vi "(SubVI)_2D_CreateFile_MultiVessel_Ver17.vi"(2 "Scanning Method":enum16{"2D", "3D"}(ring), 4 "B-scan Rep":dbl, 6 "error in":errorcluster, 7 "2D Label":string="Untitled", 8 "BD":bool=TRUE, 9 "Camera Param":T2, 10 "Galvo Param":T1, 11 "Path":path=path "C:/OCT_Data") -> (0 "error out":errorcluster, 3 "refnum out":refnum<file>)   [LabVIEW 2019]
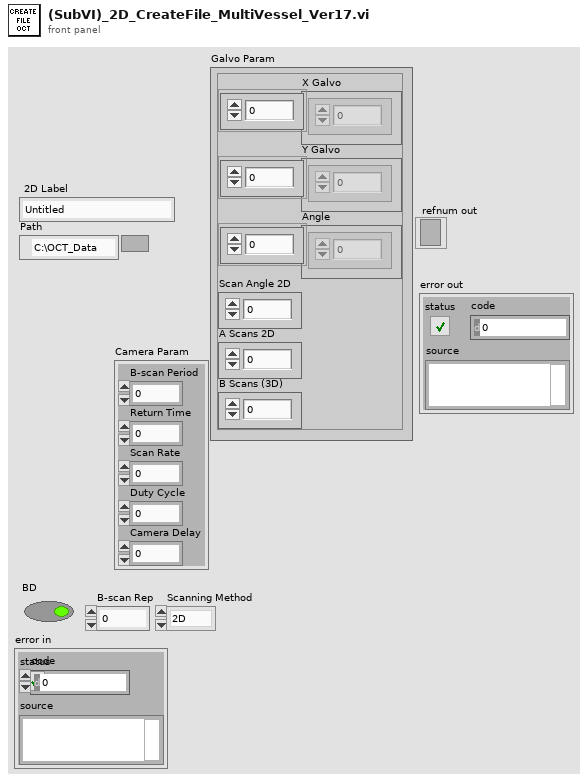
[diagram p1: front panel]
types:
  T1 = cluster{"X Galvo":dbl[], "Y Galvo":dbl[], "Angle":dbl[], "Scan Angle 2D":dbl, "A Scans 2D":u32, "B Scans (3D)":u32}
  T2 = cluster{"B-scan Period":dbl, "Return Time":dbl, "Scan Rate":dbl, "Duty Cycle":dbl, "Camera Delay":dbl}
  T3 = enum16{"big-endian, network order", "native, host order", "little-endian"}
  T4 = enum16{"open", "replace", "create", "open or create", "replace or create", "replace or create with confirmation"}
  T5 = cluster{"string":string, "string":string, "string":string, "Scan Angle 2D":dbl, "string":string, "X Galvo":dbl[], "string":string, "Y Galvo":dbl[], "string":string, "Angle":dbl[], "string":string, "Scan Angle 2D":dbl, "string":string, dbl, "string":string, dbl}
  T6 = cluster{"string":string, "B-scan Period":dbl, "string":string, "Return Time":dbl, "string":string, "Scan Rate":dbl, "string":string, "Camera Delay":dbl, "string":string, "Duty Cycle":dbl, "string":string, "Scan Rate":dbl}
  T7 = cluster{cluster{"string":string, "string":string, "string":string, "Scan Angle 2D":dbl, "string":string, "X Galvo":dbl[], "string":string, "Y Galvo":dbl[], "string":string, "Angle":dbl[], "string":string, "Scan Angle 2D":dbl, "string":string, dbl, "string":string, dbl}, cluster{"string":string, "B-scan Period":dbl, "string":string, "Return Time":dbl, "string":string, "Scan Rate":dbl, "string":string, "Camera Delay":dbl, "string":string, "Duty Cycle":dbl, "string":string, "Scan Rate":dbl}, cluster{"string":string, "B-scan Rep":dbl}, "string":string, "string":string}
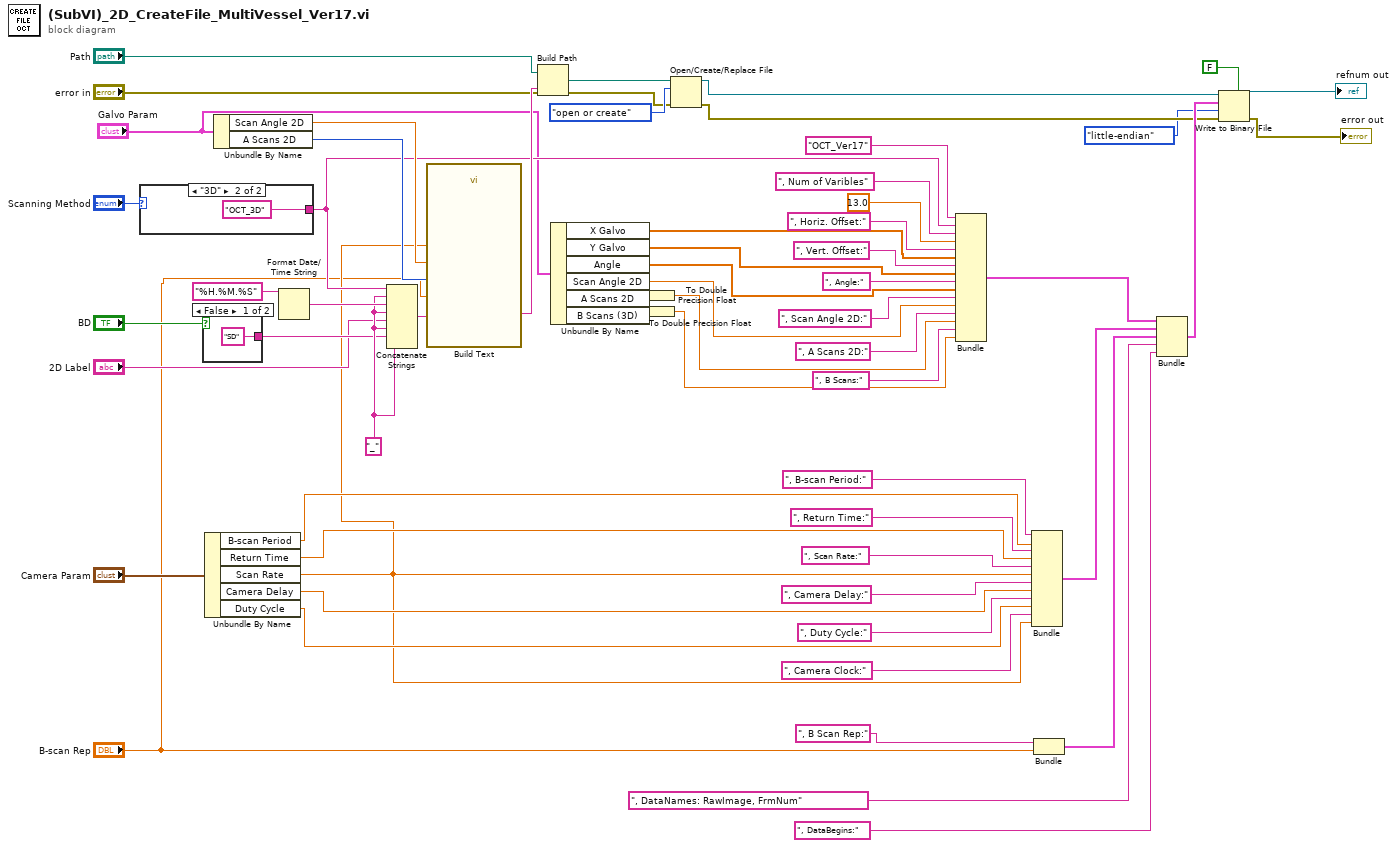
[diagram p0: block diagram]
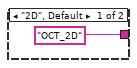
[diagram p2: hidden frame]
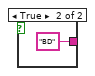
[diagram p3: hidden frame]
diagram:
  w55 = "_" ("3D Label")
  n1 = case shown="\"3D\"" "Scanning Method" {
    tunnel: ["OCT_2D" ("string") "OCT_3D" ("string")] -> w11
    frame "2D", Default {
    }
    frame "3D" {
    }
  }
  n2 = case shown="False" "BD" {
    tunnel: ["SD" ("string") "BD" ("string")] -> w53
    frame False {
    }
    frame True {
    }
  }
  n3 = Unbundle By Name("Camera Param") -> ("B-scan Period"=w9:dbl, "Return Time"=w8:dbl, "Scan Rate"=w5:dbl, "Camera Delay"=w7:dbl, "Duty Cycle"=w6:dbl)
  n4 = Unbundle By Name("Galvo Param") -> ("Scan Angle 2D"=w48:dbl, "A Scans 2D"=w52:u32)
  n5 = Format Date/Time String(time format string (%c)="%H.%M.%S") -> (date/time string=w59:string)  [unwired: 2 in]
  n6 = Concatenate Strings(w11, w55, w59, w55, "2D Label", w55, w53, w55) -> (w58:string)
  n7 = call "Build Text"("Beginning Text"=w58, "x"="B-scan Rep", "K"=w5, "SA"=w48, "A"=w52) -> ("Result"=w57:string)  [unwired: 9 in, 1 out]
  n8 = Build Path(base path="Path", name or relative path=w57) -> (appended path=w50:path)
  n9 = Unbundle By Name("Galvo Param") -> ("X Galvo"=w14:dbl[], "Y Galvo"=w13:dbl[], "Angle"=w15:dbl[], "Scan Angle 2D"=w16:dbl, "A Scans 2D"=w46:u32, "B Scans (3D)"=w22:u32)
  n10 = To Double Precision Float(number=w46) -> (double precision float=w40:dbl)
  n11 = To Double Precision Float(number=w22) -> (double precision float=w21:dbl)
  n12 = Open/Create/Replace File(file path (use dialog)=w50, error in="error in", operation (0:open)=T4."open or create") -> (refnum out=w30:refnum<file>, error out=w29:errorcluster)  [unwired: 3 in, 1 out]
  n13 = Bundle("string"="OCT_Ver17", "string"=w11, "string"=", Num of Varibles", "Scan Angle 2D"=13.0, "string"=", Horiz. Offset:", "X Galvo"=w14, "string"=", Vert. Offset:", "Y Galvo"=w13, "string"=", Angle:", "Angle"=w15, "string"=", Scan Angle 2D:", "Scan Angle 2D"=w16, "string"=", A Scans 2D:", w40, "string"=", B Scans:", w21) -> (w33:T5)  [unwired: 1 in]
  n14 = Bundle("string"=", B-scan Period:", "B-scan Period"=w9, "string"=", Return Time:", "Return Time"=w8, "string"=", Scan Rate:", "Scan Rate"=w5, "string"=", Camera Delay:", "Camera Delay"=w7, "string"=", Duty Cycle:", "Duty Cycle"=w6, "string"=", Camera Clock:", "Scan Rate"=w5) -> (w32:T6)  [unwired: 1 in]
  n15 = Bundle("string"=", B Scan Rep:", "B-scan Rep"="B-scan Rep") -> (w18:cluster{"string":string, "B-scan Rep":dbl})  [unwired: 1 in]
  n16 = Bundle(w33, w32, w18, "string"=", DataNames: RawImage, FrmNum", "string"=", DataBegins:") -> (w31:T7)  [unwired: 1 in]
  n17 = Write to Binary File(file (use dialog)=w30, data=w31, error in=w29, 5:FALSE ("prepend array or string size? (T)"), 9:T3."little-endian" ("byte order (0:big-endian, network order)")) -> (refnum out=→"refnum out":refnum<file>, error out=→"error out":errorcluster)  [unwired: 1 in, 1 out]
